vi "Set Test Complete Event.vi"(8 "error in (no error)":errorcluster, 10 "Test Complete Event":refnum<user-event>, 11 "Template Properties in":refnum<class "App Properties.lvclass">) -> (0 "error out":errorcluster, 3 "Template Properties out":refnum<class "App Properties.lvclass">)   [LabVIEW 2015]
uses:
  App Properties.lvclass
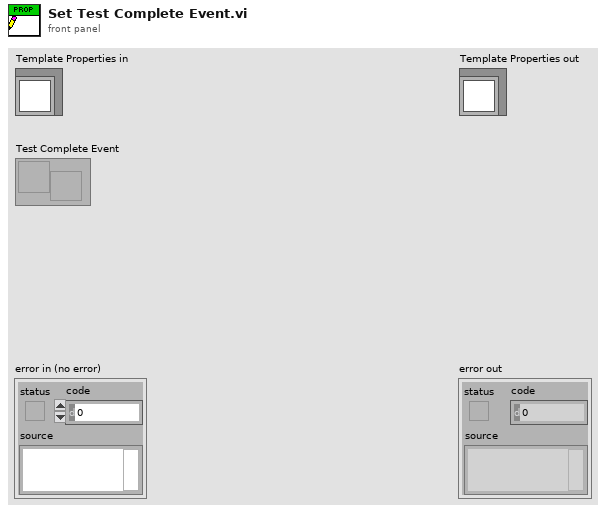
[diagram p1: front panel]
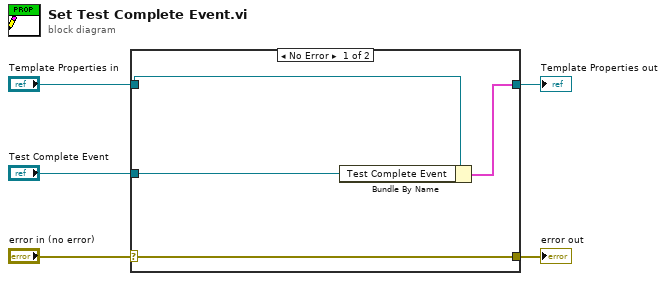
[diagram p0: block diagram]
diagram:
  n1 = case shown="No Error" "error in (no error)" {
    selector: "error in (no error)" -> [w9 w10]
    tunnel: [w9 w10] -> w4
    tunnel: [w7 w11] -> w2
    tunnel: "Template Properties in" -> [w8 w11]
    tunnel: "Test Complete Event" -> [w6 _]
    frame No Error {
      n2 = Bundle By Name(cluster=w8, "Test Complete Event"=w6) -> (w7:cluster{})
    }
    frame Error {
    }
  }
  "error out" <- w4
  "Template Properties out" <- w2
